vi "Comparison_Decision.vi"(9 "decision":dbl[](array[numeric]), 10 "SWLDA":dbl[](array[numeric]), 11 "EPR_발생_total":i16[](array[numeric])) -> (3 "selected":i32)   [LabVIEW 2014]
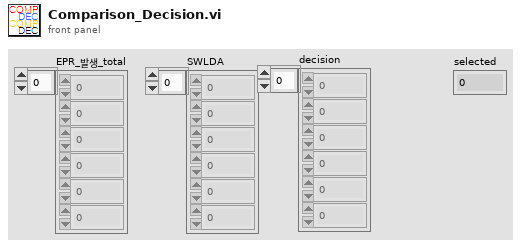
[diagram p1: front panel]
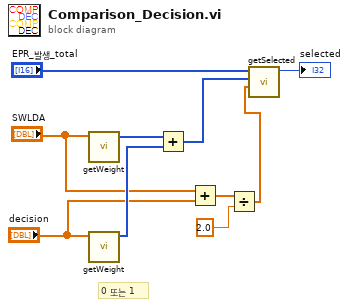
[diagram p0: block diagram]
diagram:
  # "0 또는 1"
  n1 = call "getWeight.vi"("Array"="SWLDA") -> ("Weight"=w10:i32[])  [unwired: 10 in]
  n2 = call "getWeight.vi"("Array"="decision") -> ("Weight"=w9:i32[])  [unwired: 10 in]
  n3 = Add(x=w10, y=w9) -> (x+y=w7:i32[])
  n4 = Add(x="SWLDA", y="decision") -> (x+y=w3:dbl[])
  n5 = Divide(x=w3, y=2.0) -> (x/y=w1:dbl[])
  n6 = call "getSelected.vi"("Amp"=w1, "Weight"=w7, "Predict"="EPR_발생_total") -> ("selected"=→"selected":i32)  [unwired: 8 in]
